vi "ControlPlans.vi"() -> ()   [LabVIEW 2019]
uses:
  <vilib>/Bytelabs/ByteREST/ByteRESTClass/ByteRESTBase/RESTBase.lvclass
  <vilib>/Bytelabs/ByteREST/CfgLoaders/LoaderIni/RESTLoaderIni.lvclass/RESTLoaderIni.ctl
  <vilib>/Bytelabs/ByteREST/CfgLoaders/LoaderIni/RESTLoaderIni.lvclass
  C:/Program Files (x86)/National Instruments/LabVIEW 2019/vi.lib/Bytelabs/ByteREST/CfgLoaders/LoaderBase/RESTLoaderBase.lvclass
panel:
  in  "Ini path":path
  out "error out":errorcluster
  out "Body":string
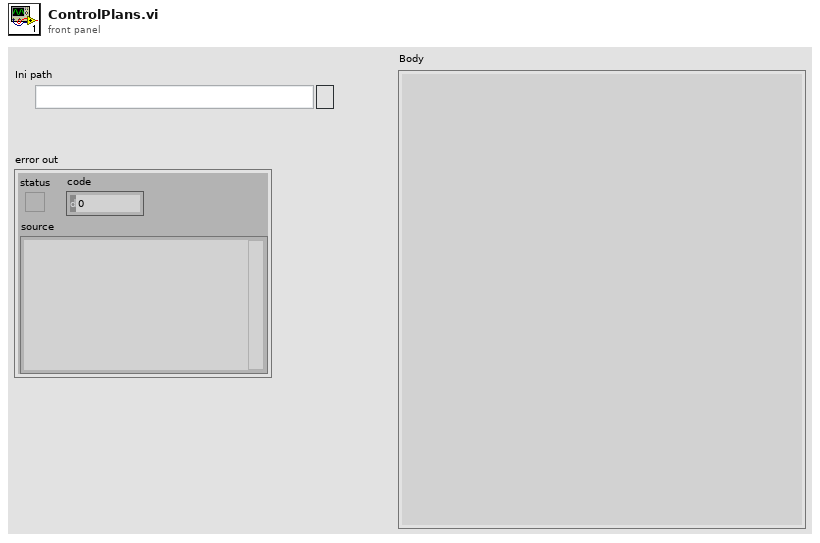
[diagram p1: front panel]
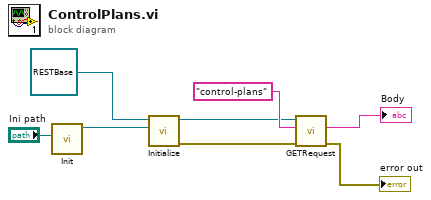
[diagram p0: block diagram]
diagram:
  n1 = call <vilib>:"Init.vi"("Ini path"="Ini path") -> ("RESTLoaderIni out"=w4:refnum<class "RESTLoaderIni.lvclass">)  [unwired: 10 in]
  n2 = call-dynamic "Initialize.vi"("RESTLoader"=w4, "REST in"=refnum<class "RESTBase.lvclass"> refnum) -> ("error out"=w5:errorcluster, "REST out"=w2:refnum<class "RESTBase.lvclass">)  [unwired: 8 in]
  n3 = call-dynamic "GETRequest.vi"("error in (no error)"=w5, "Request"="control-plans", "ByteRESTBase in"=w2) -> ("error out"=→"error out":errorcluster, "Body"=→"Body":string)  [unwired: 5 in, 2 out]
